vi "Array_singleX_multipleY.vi"(0 "graph array summary":cluster{"index":u16, "length":u16}[](array[cluster]), 1 "x-column name":string, 2 "Sort?":bool, 5 "graph file":cluster{"all rows":dbl[], "all rows":dbl[]}[](array[cluster]), 7 "col. extension.":string="_", 12 "new y-column names":string[](array[string])) -> (4 "all worksheet per file":dbl[][](array[numeric]), 6 "column names out":string, 8 "graph array":cluster{"output":dbl[], "output":dbl[]}[](array[cluster]))   [LabVIEW 2025]
panel:
  out "appended array":dbl[][](array[numeric])
  out "size(s)":i32[](array[numeric])
  out "XY Graph":cluster{"all rows":dbl[], "all rows":dbl[]}(graph)
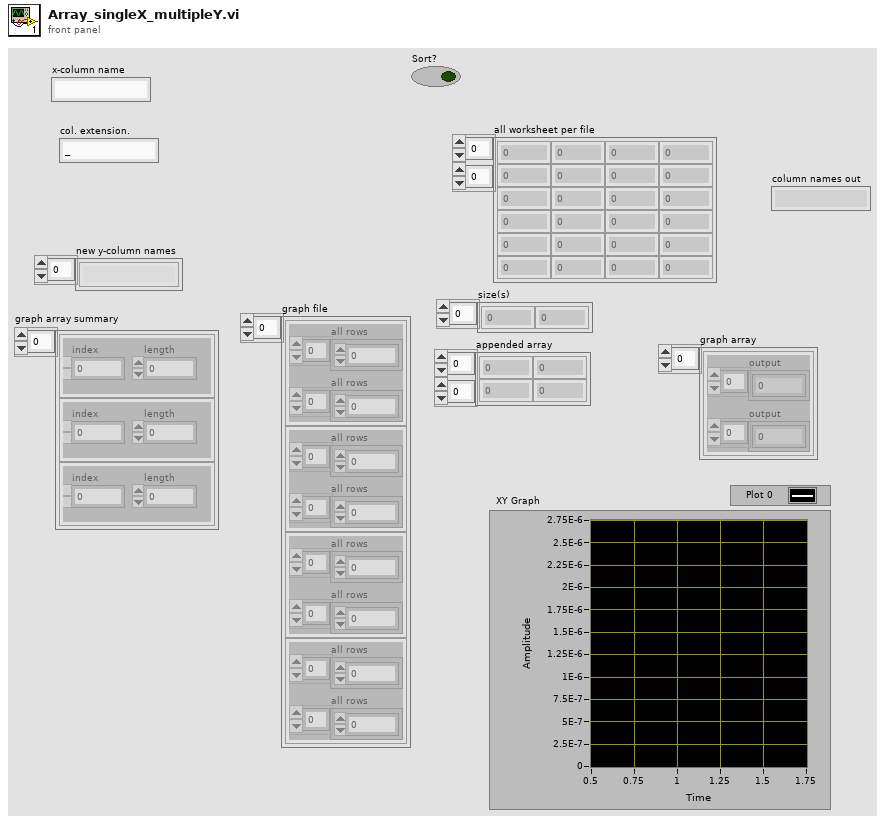
[diagram p1: front panel]
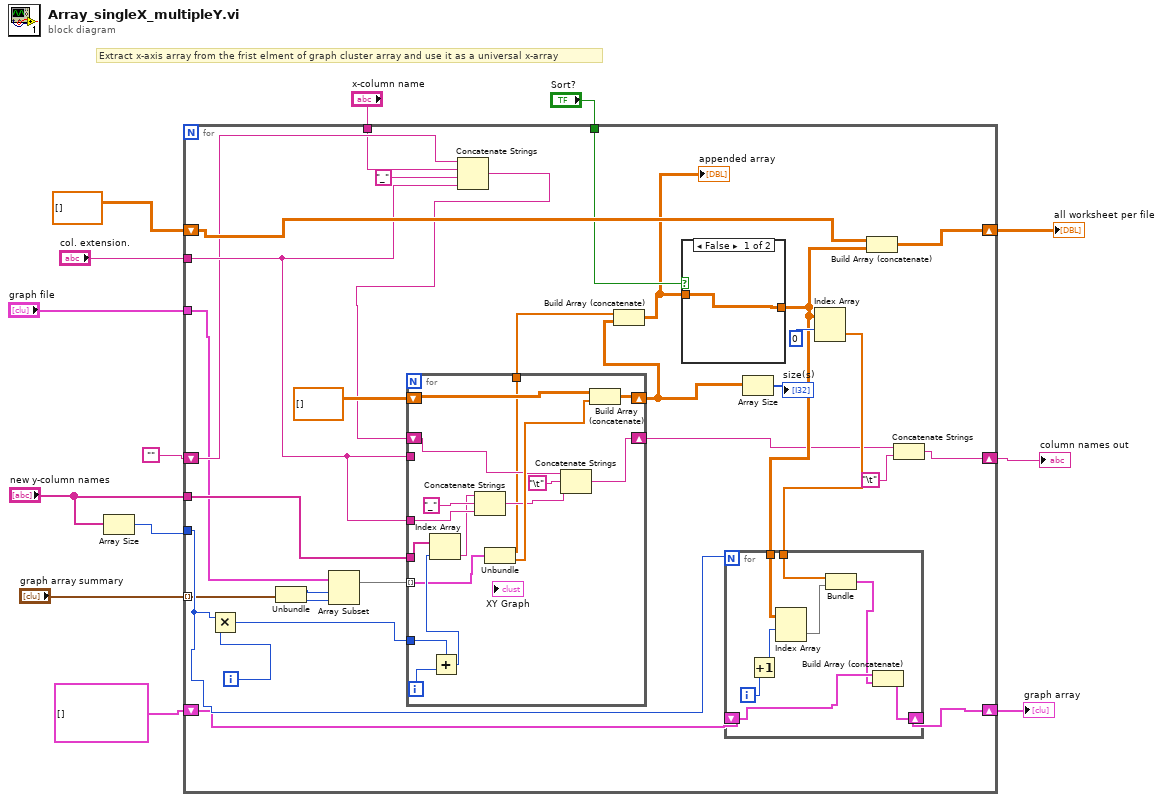
[diagram p0: block diagram]
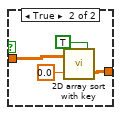
[diagram p2: hidden frame]
diagram:
  # "Extract x-axis array from the frist elment of graph cluster array and use it as a universal x-array"
  n1 = Array Size(array="new y-column names") -> (size(s)=w5:i32)
  n2 = for {
    tunnel: "col. extension." -> [w31]
    tunnel: "new y-column names" -> [w43]
    tunnel: "graph file" -> [w19]
    tunnel: w5 -> [w39]
    shift-right: [w37] -> w8
    shift-left: cluster{"all rows":sgl[], "all rows":sgl[]}[] [] ("Array 4") -> [w38]
    shift-right: [w35] -> w9
    shift-left: dbl[][] [] ("Array in") -> [w33]
    shift-right: [w28] -> w10
    shift-left: "" -> [w30]
    tunnel: "x-column name" -> [w24]
    tunnel: "Sort?" -> [w23]
    tunnel: "graph array summary" -> [w22] mode=indexing
    i -> [w26]
    n3 = Multiply(x=w39, y=w26) -> (x*y=w42:i32)
    n4 = Unbundle(w22) -> ("index"=w21:u16, "length"=w20:u16)
    n5 = Array Subset(array=w19, index=w21, length=w20) -> (w18:cluster{"all rows":dbl[], "all rows":dbl[]}[])
    n6 = Concatenate Strings(w30, w24, "_" ("string"), w31) -> (w25:string)
    n7 = for {
      tunnel: w43 -> [w61]
      tunnel: w31 -> [_]
      tunnel: w42 -> [w72]
      tunnel: w18 -> [w57] mode=indexing
      shift-right: [w68] -> w16
      shift-left: dbl[][] [] -> [w70]
      tunnel: w31 -> [w66]
      shift-right: [w63] -> w29
      shift-left: w25 -> [w64]
      tunnel: [w58] -> w17
      i -> [w71]
      n8 = Add(x=w72, y=w71) -> (x+y=w60:i32)
      n9 = Index Array(array=w61, index=w60) -> (element=w59:string)
      n10 = Concatenate Strings(w59, "_" ("string"), w66) -> (w65:string)
      n11 = Unbundle(w57) -> ("all rows"=w58:dbl[], "all rows"=w69:dbl[])
      n12 = Concatenate Strings(w64, "\t", w65) -> (w63:string)
      n13 = Build Array (concatenate)(w70, w69) -> (w68:dbl[][])
    }
    n14 = Build Array (concatenate)(w17, w16) -> (w14:dbl[][])
    "appended array" <- w14
    n15 = case shown="False" w23 {
      tunnel: w14 -> [w52 w56]
      tunnel: [w52 w53] -> w34
      frame False {
      }
      frame True {
        n16 = call "2D array sort with key.vi"("ascending"=TRUE, "key row"=0.0, "input"=w56) -> ("output"=w53:dbl[][])
      }
    }
    n17 = Array Size(array=w16) -> (size(s)=→"size(s)":i32[])
    n18 = Index Array(array=w34, index (row)=0 ("disabled index (col)")) -> (element=w40:dbl[])  [unwired: 1 in]
    n19 = for {
      N: w39 -> [_]
      tunnel: w40 -> [w51]
      tunnel: w34 -> [w49]
      shift-right: [w45] -> w37
      shift-left: w38 -> [w47]
      i -> [w50]
      n20 = Increment(x=w50) -> (x+1=w48:i32)
      n21 = Index Array(array=w49, index (row)=w48) -> (element=w44:dbl[])  [unwired: 1 in]
      n22 = Bundle("output"=w51, "output"=w44) -> (w46:cluster{"output":dbl[], "output":dbl[]})  [unwired: 1 out]
      n23 = Build Array (concatenate)(w47, w46) -> (w45:cluster{"output":dbl[], "output":dbl[]}[])
    }
    n24 = Build Array (concatenate)(w33, w34) -> (w35:dbl[][])
    n25 = Concatenate Strings(w29, "\t") -> (w28:string)
  }
  "column names out" <- w10
  "all worksheet per file" <- w9
  "graph array" <- w8
